vi "AcquireImage.vi"(8 "error in":errorcluster, 11 "Session In":T1) -> (0 "error out":errorcluster, 2 "Session Out":T1, 3 "Image":T2(plugin-control))   [LabVIEW 2017]
uses:
  <vilib>/userdefined/High Color/IMAQdx.ctl
  <vilib>/vision/driver/NI_Vision_Acquisition_Software.lvlib
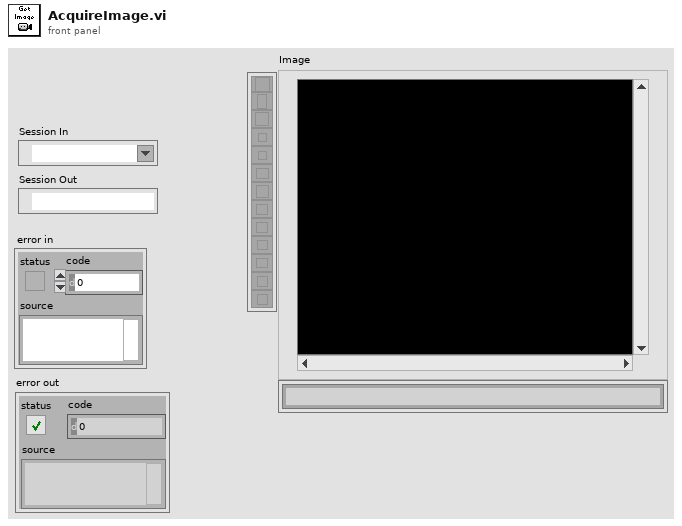
[diagram p1: front panel]
types:
  T1 = typedef "IMAQdx.ctl" = refnum<k21>
  T2 = typedef "IMAQ Image.ctl" = refnum<image>
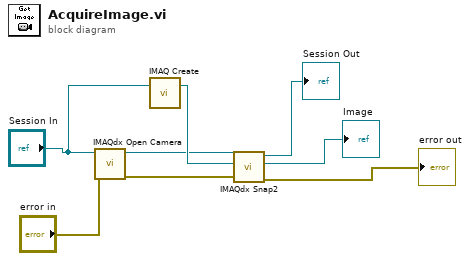
[diagram p0: block diagram]
diagram:
  n1 = call <vilib>:"IMAQdx Open Camera.vi"("error in"="error in", "Session In"="Session In") -> ("error out"=w3:errorcluster, "Session Out"=w5:T1)  [unwired: 8 in]
  n2 = call "IMAQ Create"("Image Name"="Session In") -> ("New Image"=w6:T2)  [unwired: 4 in, 1 out]
  n3 = call <vilib>:"IMAQdx Snap2.vi"("error in"=w3, "Image In"=w6, "Session In"=w5) -> ("error out"=→"error out":errorcluster, "Image Out"=→"Image":T2, "Session Out"=→"Session Out":T1)  [unwired: 6 in]
